vi "GetSerializableData_StaticCommunity.vi"(8 "error in (no error)":errorcluster, 9 "Options":T7, 10 "Data in":T1, 11 "BlueSerializable in":refnum<class "BlueSerializable.lvclass">) -> (0 "error out":errorcluster, 2 "Data out":T1, 3 "BlueSerializable out":refnum<class "BlueSerializable.lvclass">)   [LabVIEW 2020, in "BlueSerialization.lvlib" / "BlueSerializable.lvclass"]
uses:
  BlueSerializable.lvclass
  BlueSerializer/Support/GetSerializableDataCluster.ctl
  BlueSerializer/GetSerializableDataAction.ctl
  BlueSerializer/Support/GetSerializableDataClusterClass.ctl
  BlueSerializer/Support/SerializableDataGetDataAction.ctl
  BlueSerializer/ClassNameAndVersion.ctl
  <vilib>/Utility/EditLVLibs/LibVersion.ctl
  BlueSerializer/SerializeOptionsPayload.ctl
  BlueSerializer/SerializeOptions.ctl
  BlueSerializer/ClassNameCacheCluster.ctl
  BlueSerializer/ClassNameCacheMap.ctl
  BlueSerializer/ClassNameObj.ctl
  BlueSerializer/BlueSerializer.lvclass
  <vilib>/Utility/EditLVLibs/Edit LVLibs.lvlib
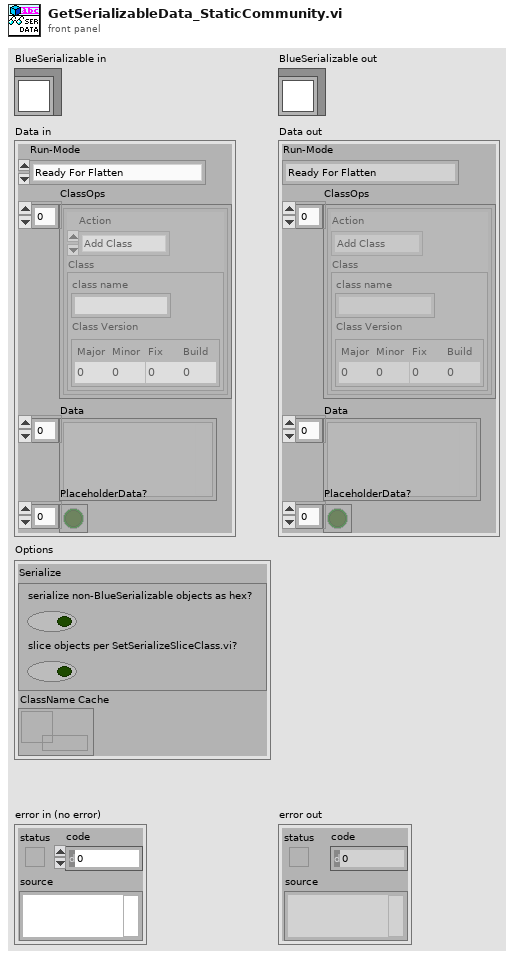
[diagram p1: front panel]
types:
  T1 = typedef "BlueSerialization.lvlib/BlueSerializer.lvclass/GetSerializableDataCluster.ctl" = cluster{"Run-Mode":T2, "ClassOps":T3[], "Data":variant[], "PlaceholderData?":bool[]}
  T2 = typedef "BlueSerialization.lvlib/BlueSerializer.lvclass/GetSerializableDataAction.ctl" = enum16{"Ready For Flatten", "Unmodified Data Access"}
  T3 = typedef "BlueSerialization.lvlib/BlueSerializer.lvclass/GetSerializableDataClusterClass.ctl" = cluster{"Action":T4, "Class":T5}
  T4 = typedef "BlueSerialization.lvlib/BlueSerializer.lvclass/SerializableDataGetDataAction.ctl" = enum16{"Add Class", "Drop Class"}
  T5 = typedef "BlueSerialization.lvlib/BlueSerializer.lvclass/ClassNameAndVersion.ctl" = cluster{"class name":string, "Class Version":T6}
  T6 = typedef "Edit LVLibs.lvlib/LibVersion.ctl" = cluster{"Major":u16, "Minor":u16, "Fix":u16, "Build":u16}
  T7 = typedef "BlueSerialization.lvlib/BlueSerializer.lvclass/SerializeOptionsPayload.ctl" = cluster{"Serialize":T8, "ClassName Cache":refnum<data-value>}
  T8 = typedef "BlueSerialization.lvlib/BlueSerializer.lvclass/SerializeOptions.ctl" = cluster{"serialize non-BlueSerializable objects as hex?":bool, "slice objects per SetSerializeSliceClass.vi?":bool}
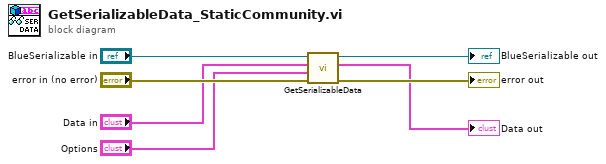
[diagram p0: block diagram]
diagram:
  n1 = call-dynamic "GetSerializableData.vi"("error in (no error)"="error in (no error)", "Options"="Options", "Data in"="Data in", "BlueSerializable in"="BlueSerializable in") -> ("error out"=→"error out":errorcluster, "Data out"=→"Data out":T1, "BlueSerializable out"=→"BlueSerializable out":refnum<class "BlueSerializable.lvclass">)  [unwired: 5 in]
